vi "Data FGV.vi"(0 "Params":T6={"Acquire?"=FALSE, "Wave Parameters"={"Frequency (Hz)"=5.0, "Phase offset (deg)"=0.0, "Vpeak (V)"=5.0, "Offset (V)"=0.0, "Waveform"=enum."Sine", "Channel"=enum."CH0"}, "Time"={"Time/Div"=0.0}} {"Time"."Time/Div" min=0.0 max=16.0 step=1.0 scale=0.0..12.0; "Wave Parameters"."Phase offset (deg)" format="%#_6p"; "Wave Parameters"."Frequency (Hz)" format="%#_6p"}, 1 "Action":T8, 5 "Data":dbl[](array[numeric]), 9 "Acquire? (Unused)":bool=TRUE, 11 "error in (no error)":errorcluster) -> (4 "Wave Parameters":T3={"Frequency (Hz)"=5.0, "Phase offset (deg)"=0.0, "Vpeak (V)"=5.0, "Offset (V)"=0.0, "Waveform"=enum."Sine", "Channel"=enum."CH0"} {"Phase offset (deg)" format="%#_6p"; "Frequency (Hz)" format="%#_6p"}, 6 "Scope Data":T7, 8 "Time":T1 {"Time/Div" min=0.0 max=16.0 step=1.0 scale=0.0..12.0}, 10 "Acquire?":bool, 15 "error out":errorcluster)   [LabVIEW 2021]
uses:
  Controls/Data FGV Action.ctl
  Communication/Scope Data.ctl
  Controls/Scope & FGen Parameters.ctl
  Program Files (x86)/National Instruments/LabVIEW 2021/ProjectTemplates/Source/myRIO/Oscilloscope/myRIO v1.1/Real-Time/Controls/Wave Parameters.ctl
  Program Files (x86)/National Instruments/LabVIEW 2021/ProjectTemplates/Source/myRIO/Oscilloscope/myRIO v1.1/Real-Time/Controls/Waveform Enum.ctl
  Program Files (x86)/National Instruments/LabVIEW 2021/ProjectTemplates/Source/myRIO/Oscilloscope/myRIO v1.1/Real-Time/Controls/Channel Selector.ctl
  Controls/Time Selector.ctl
  Controls/Time Knob.ctl
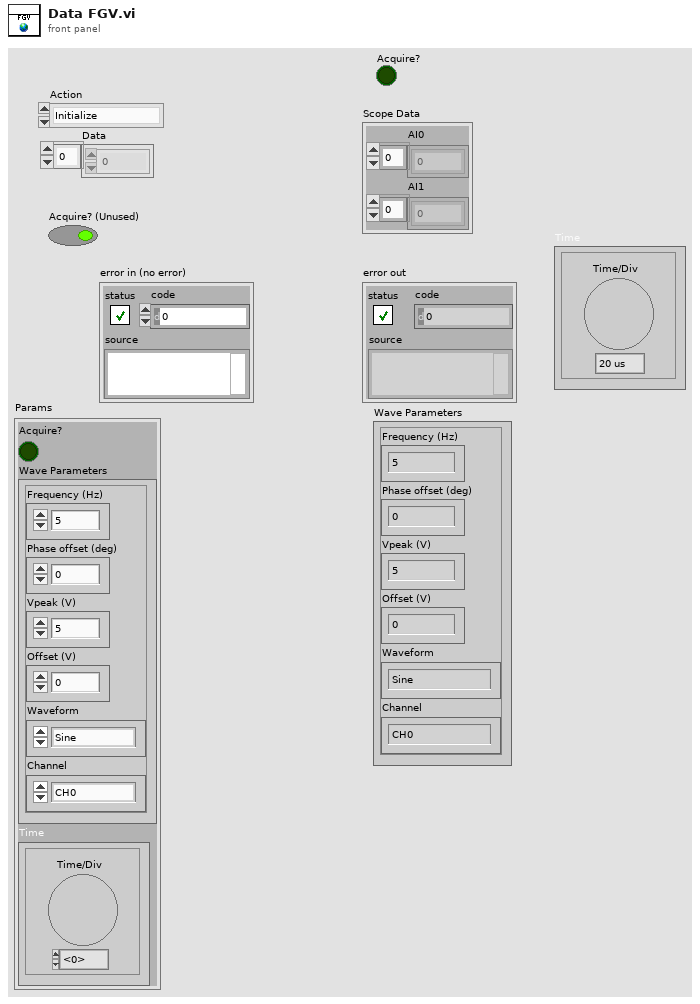
[diagram p1: front panel]
types:
  T1 = typedef "Time Selector.ctl" = cluster{"Time/Div":T2}
  T2 = typedef "Time Knob.ctl" = dbl
  T3 = typedef "Wave Parameters.ctl" = cluster{"Frequency (Hz)":dbl, "Phase offset (deg)":dbl, "Vpeak (V)":dbl, "Offset (V)":dbl, "Waveform":T4, "Channel":T5}
  T4 = typedef "Waveform Enum.ctl" = enum16{"Sine", "Square"}
  T5 = typedef "Channel Selector.ctl" = enum16{"CH0", "CH1"}
  T6 = typedef "Scope & FGen Parameters.ctl" = cluster{"Acquire?":bool, "Wave Parameters":T3, "Time":T1}
  T7 = typedef "Scope Data.ctl" = cluster{"AI0":dbl[], "AI1":dbl[]}
  T8 = typedef "Data FGV Action.ctl" = enum16{"Initialize", "Set Scope Data", "Read Scope Data", "Set FGen", "Read FGen", "Set Params"}
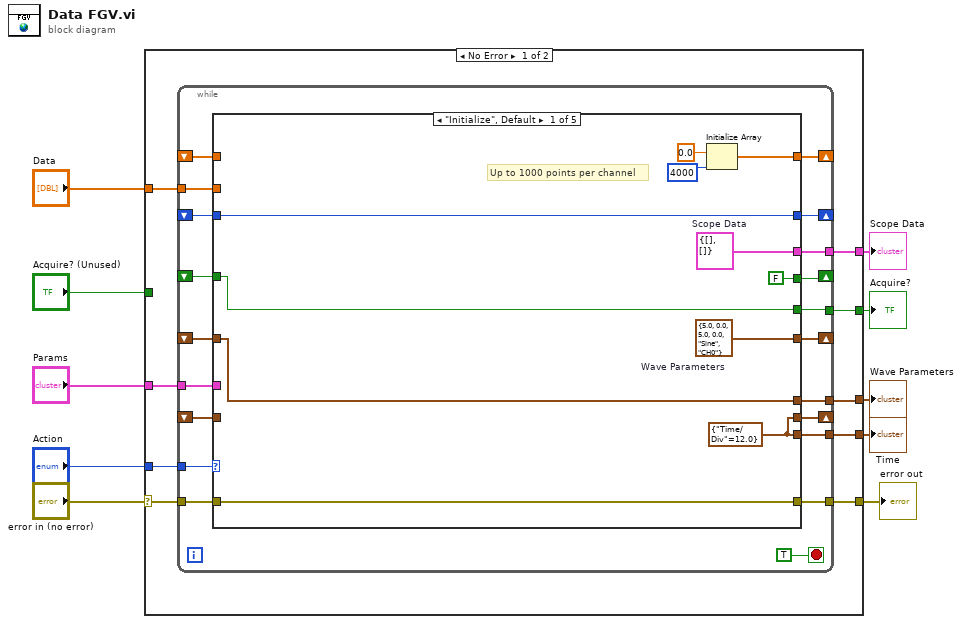
[diagram p0: block diagram]
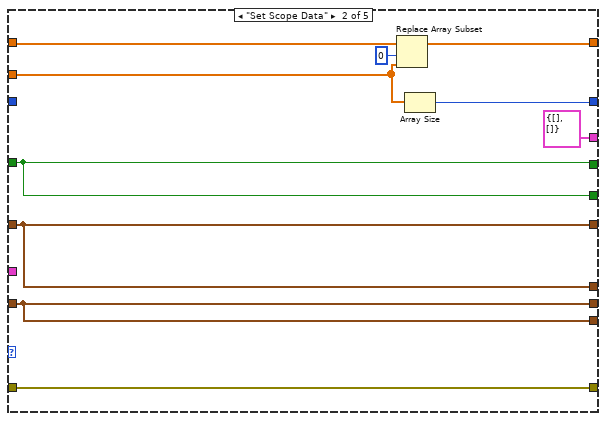
[diagram p2: hidden frame]
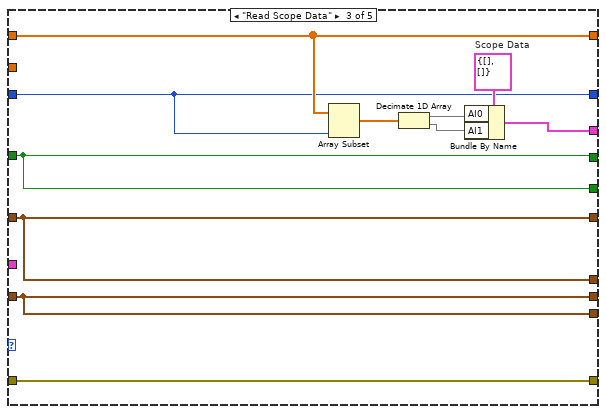
[diagram p3: hidden frame]
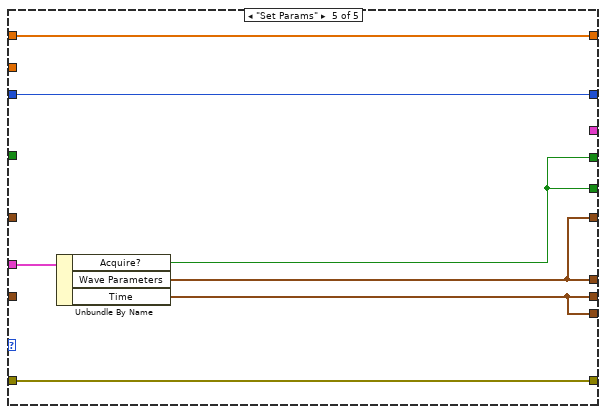
[diagram p5: hidden frame]
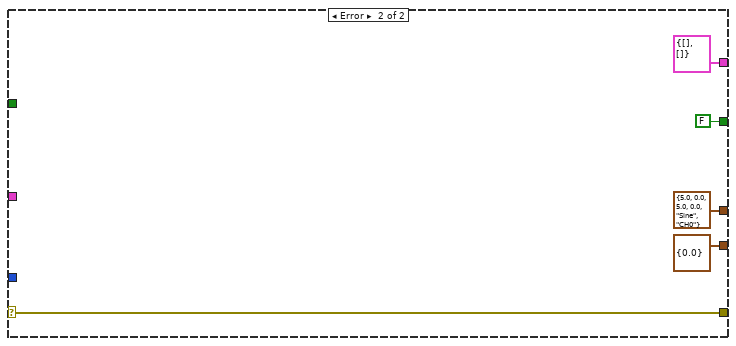
[diagram p6: hidden frame]
diagram:
  n1 = case shown="No Error" "error in (no error)" {
    selector: "error in (no error)" -> [w18 w89]
    tunnel: [w19 w89] -> w10
    tunnel: "Action" -> [w17 _]
    tunnel: "Data" -> [w16 _]
    tunnel: [w15 T7 {"AI0"=[], "AI1"=[]} ("Scope Data")] -> w6
    tunnel: "Acquire? (Unused)" -> [_ _]
    tunnel: "Params" -> [w14 _]
    tunnel: [w13 T3 {"Frequency (Hz)"=5.0, "Phase offset (deg)"=0.0, "Vpeak (V)"=5.0, "Offset (V)"=0.0, "Waveform"=enum."Sine", "Channel"=enum."CH0"} ("Wave Parameters")] -> w3
    tunnel: [w12 FALSE ("Acquire?")] -> w2
    tunnel: [w11 T1 {"Time/Div"=0.0} ("Time")] -> w1
    frame No Error {
      n2 = while {
        tunnel: w18 -> [w38]
        tunnel: [w37] -> w19
        tunnel: w17 -> [w36]
        shift-right: [w35] -> _
        shift-left: _ -> [w34]
        tunnel: w16 -> [w33]
        tunnel: [w32] -> w15
        shift-right: [w31] -> _
        shift-left: _ -> [w30]
        shift-right: [w29] -> _
        shift-left: _ -> [w28]
        tunnel: w14 -> [w27]
        tunnel: [w26] -> w13
        tunnel: [w25] -> w12
        shift-right: [w24] -> _
        shift-left: _ -> [w23]
        tunnel: [w22] -> w11
        shift-right: [w20] -> _
        shift-left: _ -> [w21]
        stop <- TRUE stop-if-true
        n3 = case shown="\"Initialize\", Default" w36 {
          tunnel: w38 -> [w50 w60 w71 w77 w84]
          tunnel: [w50 w60 w71 w77 w84] -> w37
          tunnel: [w47 w58 w63 w74 w83] -> w35
          tunnel: w34 -> [_ w59 w63 w74 w83]
          tunnel: w33 -> [_ w52 _ _ _]
          tunnel: [w46 T7 {"AI0"=[], "AI1"=[]} ("Scope Data") w67 _ _] -> w32
          tunnel: [FALSE w55 w66 w76 w80] -> w31
          tunnel: w30 -> [w43 w55 w66 w76 _]
          tunnel: [w44 w54 w65 w75 w81] -> w29
          tunnel: w28 -> [w42 w54 w65 w75 _]
          tunnel: w27 -> [_ _ _ _ w82]
          tunnel: [w42 w54 w65 w75 w81] -> w26
          tunnel: [w43 w55 w66 w76 w80] -> w25
          tunnel: [w41 w53 w64 w73 w79] -> w24
          tunnel: w23 -> [_ w53 w64 w73 _]
          tunnel: [w41 w53 w64 w73 w79] -> w22
          tunnel: w21 -> [w40 _ w61 w72 w78]
          tunnel: [w40 w51 w61 w72 w78] -> w20
          frame "Initialize", Default {
            w41 = T1 {"Time/Div"=12.0} ("Time")
            w44 = T3 {"Frequency (Hz)"=5.0, "Phase offset (deg)"=0.0, "Vpeak (V)"=5.0, "Offset (V)"=0.0, "Waveform"=enum."Sine", "Channel"=enum."CH0"}  # Wave Parameters
            w46 = T7 {"AI0"=[], "AI1"=[]}  # Scope Data
            # "Up to 1000 points per channel"
            n4 = Initialize Array(0.0, 4000 ("dimension size")) -> (w47:dbl[])
          }
          frame "Set Scope Data" {
            n5 = Replace Array Subset(array=w59, new element=w52, index=0) -> (w58:dbl[])
            n6 = Array Size(array=w52) -> (size(s)=w51:i32)
          }
          frame "Read Scope Data" {
            w70 = T7 {"AI0"=[], "AI1"=[]}  # Scope Data
            n7 = Array Subset(array=w63, length=w61) -> (w62:dbl[])  [unwired: 1 in]
            n8 = Decimate 1D Array(w62) -> (w69:dbl[], w68:dbl[])
            n9 = Bundle By Name(cluster=w70, "AI0"=w69, "AI1"=w68) -> (w67:T7)
          }
          frame "Read FGen" {
          }
          frame "Set Params" {
            n10 = Unbundle By Name(w82) -> ("Acquire?"=w80:bool, "Wave Parameters"=w81:T3, "Time"=w79:T1)
          }
        }
      }
    }
    frame Error {
    }
  }
  "error out" <- w10
  "Scope Data" <- w6
  "Wave Parameters" <- w3
  "Acquire?" <- w2
  "Time" <- w1
